vi "Read 02-03-9227.vi"() -> (3 "Array":dbl[](array[numeric]))   [LabVIEW 2018]
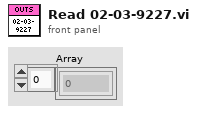
[diagram p1: front panel]
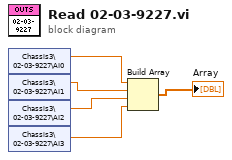
[diagram p0: block diagram]
diagram:
  n1 = shared-variable "Chassis3\\02-03-9227\\AI0"() -> (w4:dbl)  [unwired: 1 in, 1 out]
  n2 = shared-variable "Chassis3\\02-03-9227\\AI1"() -> (w3:dbl)  [unwired: 1 in, 1 out]
  n3 = shared-variable "Chassis3\\02-03-9227\\AI2"() -> (w2:dbl)  [unwired: 1 in, 1 out]
  n4 = shared-variable "Chassis3\\02-03-9227\\AI3"() -> (w1:dbl)  [unwired: 1 in, 1 out]
  n5 = Build Array(w4, w3, w2, w1) -> (→"Array":dbl[])
